vi "SPIKE-OpenMV.vi"() -> ()   [LabVIEW 2016]
uses:
  VIs/uPythonX/uPythonX.xctl
panel:
  in  "Tab Control 5":T1(tab)=enum."Spike"
  in  "LPF2Class":T2(xcontrol)={"VISA Refnum in"="ASRL12::INSTR", "Python Code"="import machine, utime, gc\n\nfrom pyb import LED\n\nred_led   = LED(1)\ngreen_led = LED(2)\nblue_led  = LED(3)\nir_led    = LED(4)\n\nclass LPF2(object):\n     def __init__(self, uartChannel, txPin, rxPin):\n          self.txPin = txPin\n          self.rxPin = rxPin\n          self.uart = machine.UART(uartChannel)\n          self.connected = False\n\n     def send_value(self,data):\n          value = (data & 0xFF)\n          payload = bytes([0xC0, value, 0xFF ^ 0xC0 ^ value])\n          size = self.uart.write(payload)\n          if not size: self.connected = False\n\n     def initialize(self):\n          self.tx = machine.Pin(self.txPin, machine.Pin.OUT)\n          self.rx = machine.Pin(self.rxPin, machine.Pin.IN)\n          self.tx.value(0)\n          utime.sleep_ms(500)\n          self.tx.value(1)\n          self.uart.init(baudrate=2400, bits=8, parity=None, stop=1)\n          self.uart.write(b'\\x00')\n          self.uart.write(b'\\x40\\x23\\x9C')\n          self.uart.write(b'\\x49\\x02\\x01\\xB5')\n          self.uart.write(b'\\x52\\x00\\xC2\\x01\\x00\\x6E')\n          self.uart.write(b'\\x5F\\x00\\x00\\x00\\x02\\x00\\x00\\x00\\x02\\xA0')\n          self.uart.write(b'\\x9A\\x00\\x4C\\x50\\x46\\x32\\x2D\\x43\\x41\\x4C\\x6E')\n          self.uart.write(b'\\x9A\\x01\\x00\\x00\\x00\\x00\\x00\\xC0\\x7F\\x44\\x9F')\n          self.uart.write(b'\\x9A\\x02\\x00\\x00\\x00\\x00\\x00\\x00\\xC8\\x42\\xED')\n          self.uart.write(b'\\x9A\\x03\\x00\\x00\\x00\\x00\\x00\\xC0\\x7F\\x44\\x9D')\n          self.uart.write(b'\\x92\\x04\\x52\\x41\\x57\\x00\\x2D')\n          self.uart.write(b'\\x8A\\x05\\x10\\x00\\x60')\n          self.uart.write(b'\\x92\\x80\\x03\\x01\\x03\\x00\\xEC')\n          utime.sleep_ms(5)\n          #  print(uart.read(uart.any()))\n          self.uart.write(b'\\xA1\\x00\\x4C\\x50\\x46\\x32\\x2D\\x43\\x4F\\x55\\x4E\\x54\\x00\\x00\\x00\\x00\\x00\\x00\\x58')\n          self.uart.write(b'\\x99\\x01\\x00\\x00\\x00\\x00\\x00\\x00\\xC8\\x42\\xED')\n          self.uart.write(b'\\x99\\x02\\x00\\x00\\x00\\x00\\x00\\x00\\xC8\\x42\\xEE')\n          self.uart.write(b'\\x99\\x03\\x00\\x00\\x00\\x00\\x00\\x00\\xC8\\x42\\xEF')\n          self.uart.write(b'\\x91\\x04\\x43\\x4E\\x54\\x00\\x33')\n          self.uart.write(b'\\x89\\x05\\x10\\x00\\x63')\n          self.uart.write(b'\\x91\\x80\\x01\\x02\\x04\\x00\\xE9')\n          utime.sleep_ms(5)\n          # print(uart.read(uart.any()))\n          self.uart.write(b'\\xA0\\x00\\x4C\\x50\\x46\\x32\\x2D\\x44\\x45\\x54\\x45\\x43\\x54\\x00\\x00\\x00\\x00\\x00\\x1D')\n          self.uart.write(b'\\x98\\x01\\x00\\x00\\x00\\x00\\x00\\x00\\x20\\x41\\x07')\n          self.uart.write(b'\\x98\\x02\\x00\\x00\\x00\\x00\\x00\\x00\\xC8\\x42\\xEF')\n          self.uart.write(b'\\x98\\x03\\x00\\x00\\x00\\x00\\x00\\x00\\x20\\x41\\x05')\n          self.uart.write(b'\\x80\\x04\\x00\\x7B')\n          self.uart.write(b'\\x88\\x05\\x10\\x00\\x62')\n          self.uart.write(b'\\x90\\x80\\x01\\x00\\x03\\x00\\xED')\n          utime.sleep_ms(5)\n          # print(uart.read(uart.any()))\n          self.uart.write(b'\\x04')  \n          # wait for ACK\n          starttime = utime.time()\n          currenttime = starttime\n          while (currenttime-starttime) < 2000:\n               utime.sleep_ms(5)\n               data = self.uart.read(self.uart.any())\n               if data.find(b'\\x04') >= 0:\n                    self.connected = True\n                    currenttime = starttime+3000   # stop the loop\n               else:\n                    currenttime = utime.time()\n          # pull pin low\n          self.uart.deinit()\n          self.tx = machine.Pin(self.txPin, machine.Pin.OUT)\n          self.tx.value(0)\n          utime.sleep_ms(10)\n          #change baudrate\n          self.uart.init(baudrate=115200, bits=8, parity=None, stop=1)"}
  in  "ToSpike":T2(xcontrol)={"VISA Refnum in"="ASRL12::INSTR", "Python Code"="import LPF2Class\n\n# loop from -10 to 10\ni=0\nred_led.on()\nlpf2 = LPF2Class.LPF2(1, 'P1', 'P0')    # OpenMV\nlpf2.initialize()\n\nwhile True:\n     if not lpf2.connected:\n          red_led.on()\n          utime.sleep(1)\n          lpf2.initialize()\n     else:\n          red_led.off()\n          while lpf2.connected:\n               gc.collect()\n               lpf2.send_value(i)\n               i += 1\n               # print(lpf2.connected)\n               if i > 10: i=-10\n               utime.sleep_ms(200)\n"}
  in  "Line":T2(xcontrol)={"VISA Refnum in"="ASRL12::INSTR", "Python Code"="import LPF2Class\nimport sensor, image, time\n\nenable_lens_corr = False # turn on for straighter lines...\n\nsensor.reset()\nsensor.set_pixformat(sensor.RGB565) # grayscale is faster\nsensor.set_framesize(sensor.QQVGA)\nsensor.skip_frames(time = 2000)\n\nmin_degree = 0\nmax_degree = 179\n\n\nred_led.on()\nlpf2 = LPF2Class.LPF2(1, 'P1', 'P0')    # OpenMV\nlpf2.connected = True\n#lpf2.initialize()\n\nwhile True:\n     img = sensor.snapshot()\n     if enable_lens_corr: img.lens_corr(1.8) # for 2.8mm lens...\n          \n     if not lpf2.connected:\n          red_led.on()\n          utime.sleep(1)\n          lpf2.initialize()\n     else:\n          red_led.off()\n          while lpf2.connected:\n               gc.collect()\n               rawLines = img.find_lines(threshold = 1000, theta_margin = 25, rho_margin = 25)\n               averageAngle = 0\n               for line in rawLines:\n                    if (min_degree <= line.theta()) and (line.theta() <= max_degree):\n                         img.draw_line(line.line(), color = (255, 0, 0))\n                         averageAngle + = line.theta()\n               value = averageAngle / len(rawLines)\n\n               lpf2.send_value(value)\n               print(value)\n               utime.sleep_ms(200)\n"}
  in  "SimpleTest":T2(xcontrol)={"VISA Refnum in"="ASRL73::INSTR", "Python Code"="import hub,utime\n\nhub.port.B.info()\n\n# if info comes back with None - then you have to restart the pybaord\n\nwhile True:\n     try:\n          value = hub.port.B.device.get()[0]\n          # print(value)\n          hub.display.show(str(value))\n          utime.sleep(0.2)\n     except:\n          utime.sleep(1)\n"}
  # "Rx\nTx"
  # "VIn\nGND"
  # "https://en.wikipedia.org/wiki/Hough_transform"
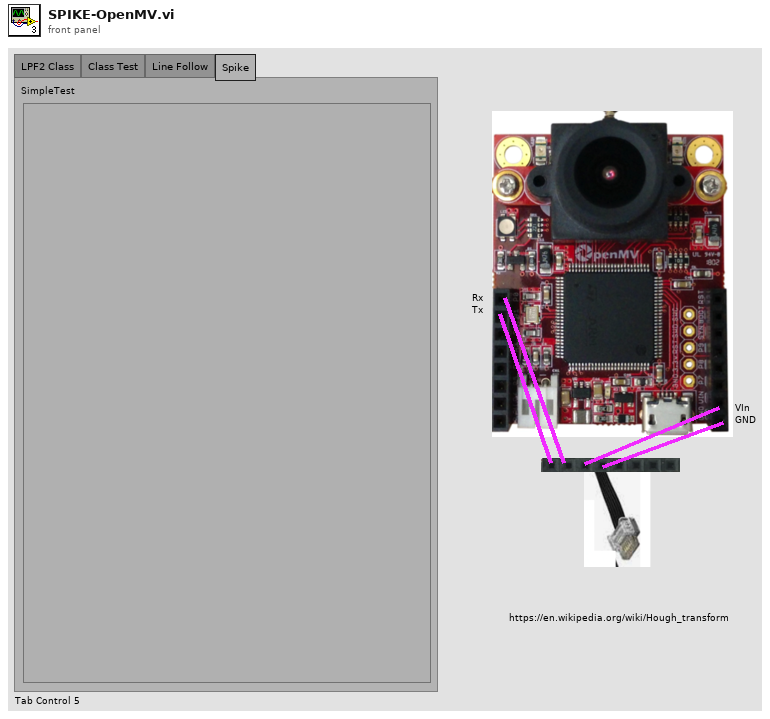
[diagram p1: front panel]
types:
  T1 = enum32{"LPF2 Class", "Class Test", "Line Follow", "Spike"}
  T2 = cluster{"VISA Refnum in":refnum<visa-resource-name>, "Python Code":string}
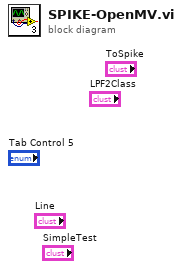
[diagram p0: block diagram]
diagram:
